vi "Dropdown - Event Timeout.vi"(0 "Table Ref":refnum<vi>, 7 "Dropdown Bundle In":T2) -> (8 "Dropdown Bundle Out":T2)   [LabVIEW 2013]
uses:
  <vilib>/Utility/miscctls.llb/LVRowAndColumnTypeDef.ctl
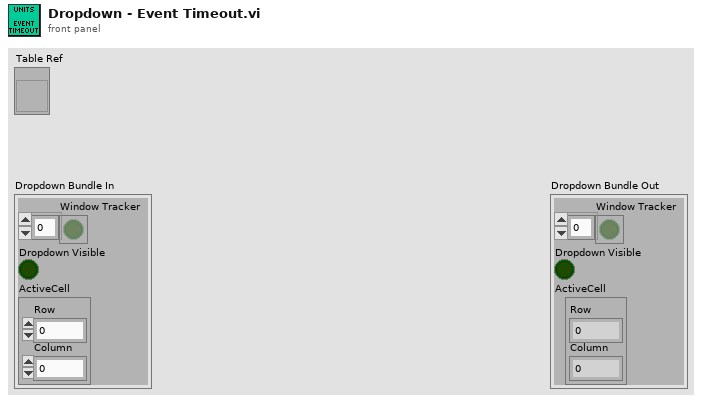
[diagram p1: front panel]
types:
  T1 = typedef "LVRowAndColumnTypeDef.ctl" = cluster{"Row":i32, "Column":i32}
  T2 = cluster{"Window Tracker":bool[], "Dropdown Visible":bool, "ActiveCell":T1}
  T3 = enum16{"Set Abbreviations", "Set Engine Mode", "Set Enum Position", "Get Abbreviation", "Write Abbreviation", "Read Enum Position", "Read Engine Mode", "Read Abbreviations", "Engine Started", "Check Engine", "Init Global", "Set Cursor", "Read Cursor"}
  T4 = enum16{"Idle", "Reveal Dropdown", "Hide FP", "Set Options"}
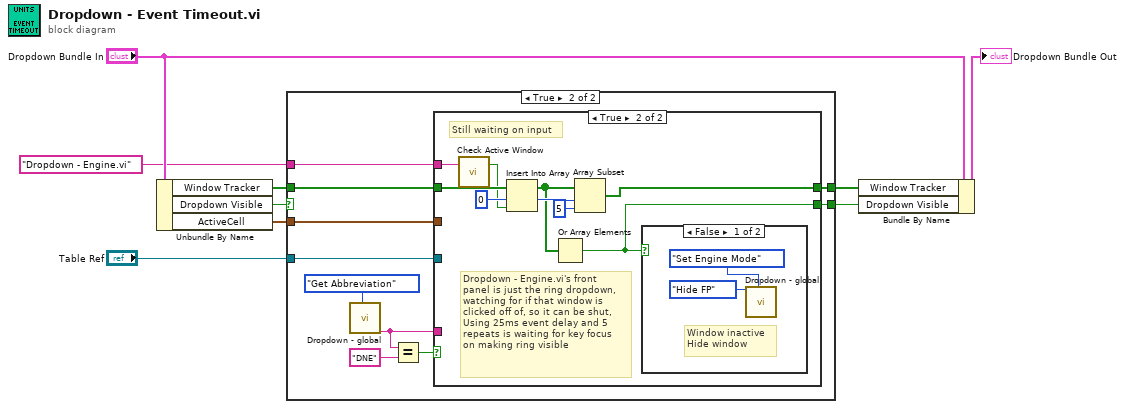
[diagram p0: block diagram]
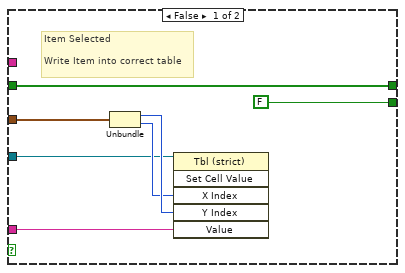
[diagram p3: hidden frame]
diagram:
  n1 = Unbundle By Name("Dropdown Bundle In") -> ("Window Tracker"=w7:bool[], "Dropdown Visible"=w8:bool, "ActiveCell"=w9:T1)
  n2 = case shown="True" w8 {
    selector: w8 -> [w11 _]
    tunnel: [w11 w19] -> w6
    tunnel: w9 -> [_ w17]
    tunnel: w7 -> [w10 w16]
    tunnel: [w10 w15] -> w3
    tunnel: "Table Ref" -> [_ w13]
    tunnel: "Dropdown - Engine.vi" ("Filename") -> [_ w12]
    frame False {
      # "Dropdown not visible\n\nNot waiting on action"
    }
    frame True {
      n3 = call "Dropdown - global.vi"("Global Mode"=T3."Get Abbreviation") -> ("Abbr Out"=w18:string)  [unwired: 10 in, 8 out]
      n4 = Equal?(x=w18, y="DNE") -> (x = y?=w20:bool)
      n5 = case shown="True" w20 {
        tunnel: [FALSE w30] -> w19
        tunnel: w18 -> [w26 _]
        tunnel: w17 -> [w25 _]
        tunnel: w16 -> [w23 w36]
        tunnel: [w23 w33] -> w15
        tunnel: w13 -> [w22 _]
        tunnel: w12 -> [_ w29]
        frame False {
          # "Item Selected\n\nWrite Item into correct table"
          n6 = Unbundle(w25) -> ("Row"=w28:i32, "Column"=w27:i32)
          n7 = invoke on="Invoke Node" class="Tbl (strict)" method="Set Cell Value"(reference=w22, "X Index"=w27, "Y Index"=w28, "Value"=w26) -> ()  [unwired: 2 in, 6 out]
        }
        frame True {
          w35 = 0 ("index")
          # "Dropdown - Engine.vi's front\npanel is just the ring dropdown,\nwatching for if that window is\nclicked off of, so it can be shut,\nUsing 25ms event delay and 5\nrepeats is waiting for key focus\non making ring visible"
          # "Still waiting on input"
          n8 = call "Check Active Window.vi"("Filename"=w29) -> ("Active Window"=w31:bool)  [unwired: 2 in]
          n9 = Insert Into Array(array=w36, index=w35, new element=w31) -> (w32:bool[])
          n10 = Or Array Elements(Boolean array=w32) -> (logical OR=w30:bool)
          n11 = Array Subset(array=w32, index=w35, length=5) -> (w33:bool[])
          n12 = case shown="False" w30 {
            frame False {
              # "Window inactive\nHide window"
              n13 = call "Dropdown - global.vi"("Engine Mode In"=T4."Hide FP", "Global Mode"=T3."Set Engine Mode") -> ()  [unwired: 9 in, 9 out]
            }
            frame True {
              # "Window still active"
            }
          }
        }
      }
    }
  }
  n14 = Bundle By Name(cluster="Dropdown Bundle In", "Window Tracker"=w3, "Dropdown Visible"=w6) -> (→"Dropdown Bundle Out":T2)
